vi "Home Stage.vi"(8 "error in (no error)":errorcluster, 11 "2-Axis Stage in":refnum<class "XY Stage Process.lvclass">) -> (0 "error out":errorcluster, 3 "2-Axis Stage out":refnum<class "XY Stage Process.lvclass">)   [LabVIEW 2022 SP3, in "XY Stage Process.lvlib" / "XY Stage Process.lvclass"]
uses:
  XY Stage Process.lvclass
  Process Framework/Process State Data/Process State Data.lvclass
  Axis Objects/iMotion Controller/iMotion Controller.lvclass
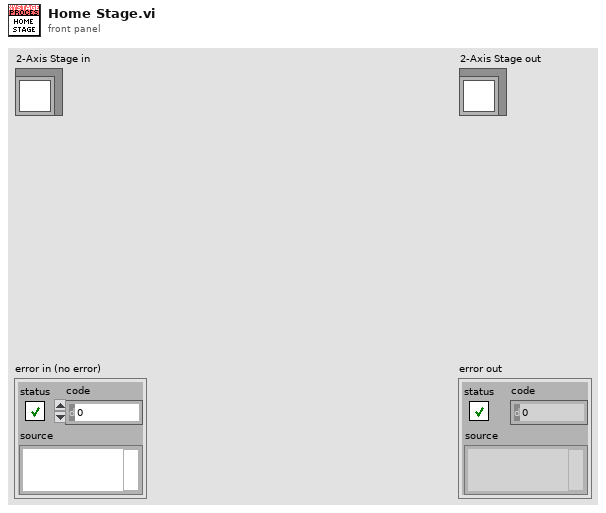
[diagram p1: front panel]
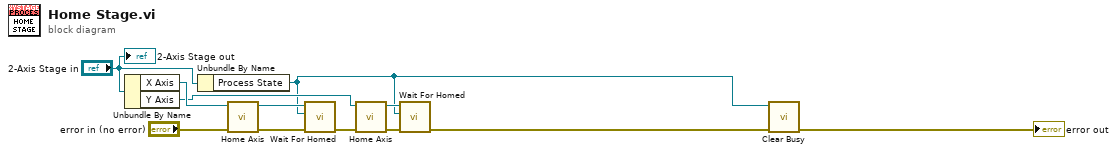
[diagram p0: block diagram]
diagram:
  n1 = Unbundle By Name("2-Axis Stage in") -> ("X Axis"=w12:refnum<class "iMotion Controller.lvclass">, "Y Axis"=w6:refnum<class "iMotion Controller.lvclass">)
  n2 = Unbundle By Name("2-Axis Stage in") -> ("Process State"=w1:refnum<data-value>)
  n3 = call-dynamic "Home Axis.vi"("error in (no error)"="error in (no error)", "iMotion Controller in"=w12) -> ("error out"=w8:errorcluster, "iMotion Controller out"=w9:refnum<class "iMotion Controller.lvclass">)  [unwired: 8 in]
  n4 = call "Wait For Homed.vi"("error in (no error)"=w8, "Process State"=w1, "iMotion Controller in"=w9) -> ("error out"=w5:errorcluster)  [unwired: 8 in]
  n5 = call-dynamic "Home Axis.vi"("error in (no error)"=w5, "iMotion Controller in"=w6) -> ("error out"=w3:errorcluster, "iMotion Controller out"=w4:refnum<class "iMotion Controller.lvclass">)  [unwired: 8 in]
  n6 = call "Wait For Homed.vi"("error in (no error)"=w3, "Process State"=w1, "iMotion Controller in"=w4) -> ("error out"=w2:errorcluster)  [unwired: 8 in]
  n7 = call "Clear Busy.vi"("error in (no error)"=w2, "Process State"=w1) -> ("error out"=→"error out":errorcluster)  [unwired: 8 in, 1 out]
  "2-Axis Stage out" <- "2-Axis Stage in"
